vi "Match_Linear.vi"(0 "환산단위(보정값)":string, 3 "절대값?":bool, 4 "기준기명":string, 5 "교정(T) 보정(F)":bool=TRUE, 6 "열팽창계수(etc)":string="0", 7 "0보다 작음?":bool, 8 "환산단위(불확도)":string="μm", 9 "Cal STD in":string[][](array[string]), 10 "환산단위(교정값)":string, 11 "Condition Default":string[][](array[string])) -> (1 "Cal STD out":string[][](array[string]), 2 "Data out":string[][](array[string]))   [LabVIEW 2020]
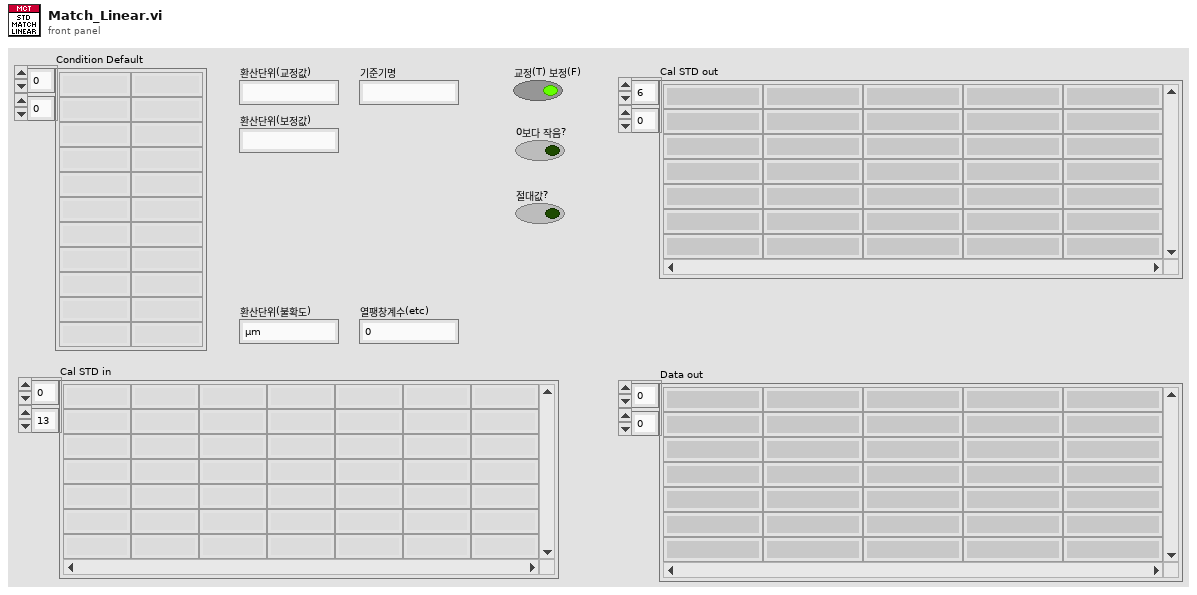
[diagram p1: front panel]
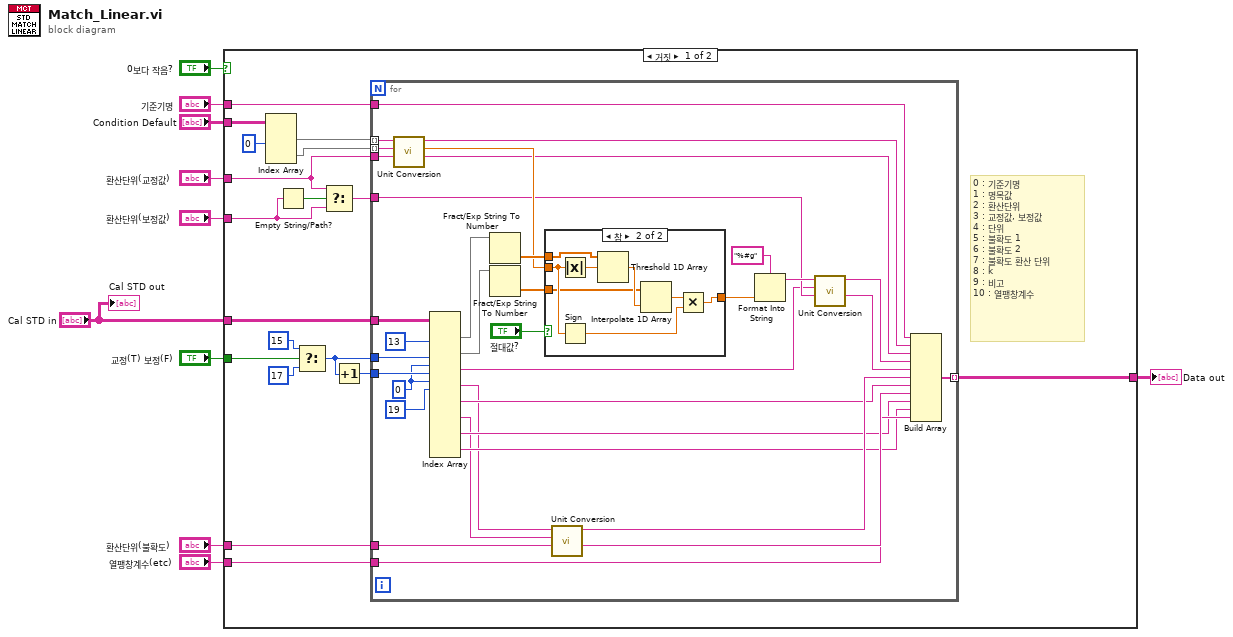
[diagram p0: block diagram]
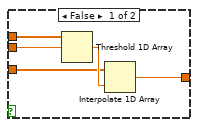
[diagram p2: hidden frame]
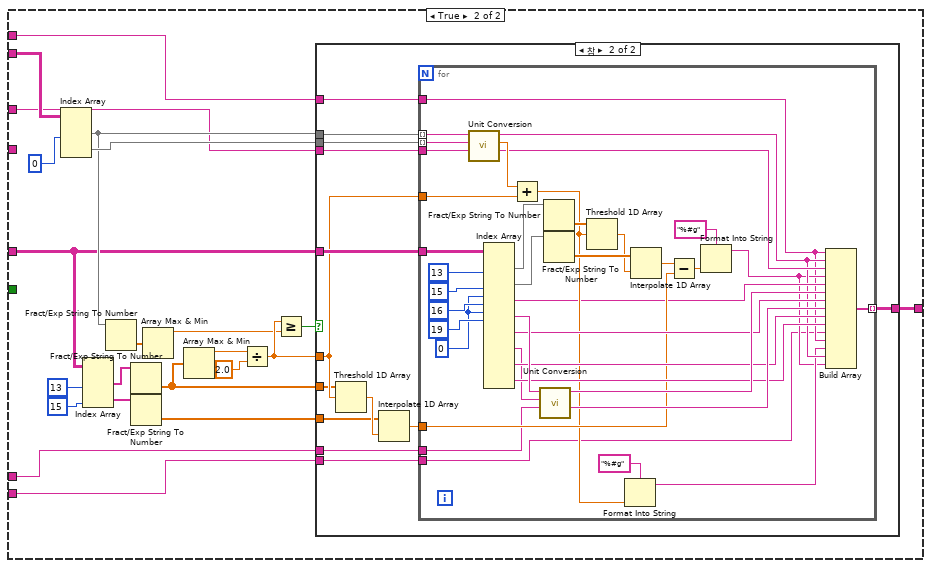
[diagram p3: hidden frame]
diagram:
  n1 = case shown="거짓" "0보다 작음?" {
    tunnel: "기준기명" -> [w28 w85]
    tunnel: "Cal STD in" -> [w27 w78]
    tunnel: "환산단위(교정값)" -> [w13 w77]
    tunnel: [w26 w88] -> w8
    tunnel: "환산단위(불확도)" -> [w25 w80]
    tunnel: "열팽창계수(etc)" -> [w24 w79]
    tunnel: "교정(T) 보정(F)" -> [w23 _]
    tunnel: "Condition Default" -> [w17 w81]
    tunnel: "환산단위(보정값)" -> [w12 _]
    frame False {
      # "0 : 기준기명\n1 : 명목값\n2 : 환산단위\n3 : 교정값, 보정값\n4 : 단위\n5 : 불확도 1\n6 : 불확도 2\n7 : 불확도 환산 단위\n8 : k\n9 : 비고\n10 : 열팽창계수"
      n2 = Index Array(array=w17, index (col) #1=0 ("비활성화된 인덱스 (열)")) -> (element #1=w16:string[], element #2=w15:string[])  [unwired: 3 in]
      n3 = Empty String/Path?(string/path=w12) -> (empty?=w14:bool)
      n4 = Select(t=15 ("인덱스 (행)"), s=w23, f=17 ("인덱스 (행)")) -> (s? t:f=w20:i32)
      n5 = Select(t=w13, s=w14, f=w12) -> (s? t:f=w11:string)
      n6 = Increment(x=w20) -> (x+1=w19:i32)
      n7 = for {
        tunnel: w27 -> [w63]
        tunnel: w16 -> [w57] mode=indexing
        tunnel: [w62] -> w26 mode=indexing
        tunnel: w15 -> [w56] mode=indexing
        tunnel: w13 -> [w55]
        tunnel: w25 -> [w54]
        tunnel: w28 -> [w53]
        tunnel: w24 -> [w48]
        tunnel: w20 -> [w45]
        tunnel: w19 -> [w44]
        tunnel: w11 -> [w31]
        w43 = 0 ("인덱스 (열)")
        n8 = call "Unit Conversion.vi"("환산단위"=w55, "입력단위"=w56, "입력값"=w57) -> ("환산단위"=w32:string, "환산값 (DBL)"=w60:dbl, "환산값 (string)"=w52:string)  [unwired: 3 in, 3 out]
        n9 = Index Array(array=w63, index (col) #1=13 ("인덱스 (행)"), index (col) #2=w45, index (row) #3=w43, index (col) #3=w44, index (row) #4=w43, index (col) #4=19 ("비활성화된 인덱스 (열)")) -> (element #1=w58:string[], element #2=w40:string[], element #3=w30:string, element #4=w36:string, element #5=w50:string, element #6=w35:string, element #7=w47:string, element #8=w46:string)  [unwired: 10 in]
        n10 = Fract/Exp String To Number(string=w58) -> (number=w61:dbl[])  [unwired: 3 in, 1 out]
        n11 = Fract/Exp String To Number(string=w40) -> (number=w39:dbl[])  [unwired: 3 in, 1 out]
        n12 = case shown="참" "절대값?" {
          tunnel: w61 -> [w68 w71]
          tunnel: w60 -> [w66 w72]
          tunnel: w39 -> [w65 w70]
          tunnel: [w64 w69] -> w37
          frame False {
            n13 = Threshold 1D Array(2:w66, 3:w68) -> (0:w67:dbl)  [unwired: 1 in]
            n14 = Interpolate 1D Array(1:w67, 2:w65) -> (0:w64:dbl)
          }
          frame True {
            n15 = Absolute Value(x=w72) -> (abs(x)=w76:dbl)
            n16 = Sign(1:w72) -> (0:w75:dbl)
            n17 = Threshold 1D Array(2:w76, 3:w71) -> (0:w74:dbl)  [unwired: 1 in]
            n18 = Interpolate 1D Array(1:w74, 2:w70) -> (0:w73:dbl)
            n19 = Multiply(x=w73, y=w75) -> (x*y=w69:dbl)
          }
        }
        n20 = call "Unit Conversion.vi"("환산단위"=w54, "입력단위"=w35, "입력값"=w36) -> ("환산단위"=w49:string, "환산값 (string)"=w51:string)  [unwired: 3 in, 4 out]
        n21 = Format Into String(format string="%#g" ("포맷 문자열"), w37) -> (resulting string=w34:string)  [unwired: 2 in, 1 out]
        n22 = call "Unit Conversion.vi"("환산단위"=w31, "입력단위"=w30, "입력값"=w34) -> ("환산단위"=w29:string, "환산값 (string)"=w33:string)  [unwired: 3 in, 4 out]
        n23 = Build Array(w53, w52, w32, w33, w29, w51, w50, w49, w47, w46, w48) -> (w62:string[])
      }
    }
    frame True {
      n24 = Index Array(array=w81, index (col) #1=0 ("비활성화된 인덱스 (열)")) -> (element #1=w82:string[], element #2=w83:string[])  [unwired: 3 in]
      n25 = Index Array(array=w78, index (col) #1=13 ("인덱스 (행)"), index (col) #2=15 ("인덱스 (행)")) -> (element #1=w91:string[], element #2=w92:string[])  [unwired: 2 in]
      n26 = Fract/Exp String To Number(string=w82) -> (number=w87:dbl[])  [unwired: 3 in, 1 out]
      n27 = Fract/Exp String To Number(string=w91) -> (number=w94:dbl[])  [unwired: 3 in, 1 out]
      n28 = Fract/Exp String To Number(string=w92) -> (number=w93:dbl[])  [unwired: 3 in, 1 out]
      n29 = Array Max & Min(array=w87) -> (max value=w86:dbl)  [unwired: 3 out]
      n30 = Array Max & Min(array=w94) -> (max value=w95:dbl)  [unwired: 3 out]
      n31 = Divide(x=w95, y=2.0) -> (x/y=w98:dbl)
      n32 = Greater Or Equal?(x=w98, y=w86) -> (x >= y?=w97:bool)
      n33 = case shown="참" w97 {
        tunnel: [_ w111] -> w88
        tunnel: w83 -> [_ w110]
        tunnel: w82 -> [_ w109]
        tunnel: w78 -> [_ w108]
        tunnel: w93 -> [_ w106]
        tunnel: w98 -> [_ w105]
        tunnel: w94 -> [_ w103]
        tunnel: w77 -> [_ w102]
        tunnel: w85 -> [_ w101]
        tunnel: w80 -> [_ w100]
        tunnel: w79 -> [_ w99]
        frame False {
        }
        frame True {
          n34 = Threshold 1D Array(2:w105, 3:w103) -> (0:w107:dbl)  [unwired: 1 in]
          n35 = Interpolate 1D Array(1:w107, 2:w106) -> (0:w104:dbl)
          n36 = for {
            tunnel: w108 -> [w149]
            tunnel: w109 -> [w146] mode=indexing
            tunnel: w110 -> [w145] mode=indexing
            tunnel: [w144] -> w111 mode=indexing
            tunnel: w105 -> [w131]
            tunnel: w104 -> [w129]
            tunnel: w102 -> [w125]
            tunnel: w101 -> [w114]
            tunnel: w100 -> [w113]
            tunnel: w99 -> [w112]
            w119 = 0 ("인덱스 (열)")
            n37 = call "Unit Conversion.vi"("환산단위"=w125, "입력단위"=w145, "입력값"=w146) -> ("환산단위"=w126:string, "환산값 (DBL)"=w139:dbl, "환산값 (string)"=w117:string)  [unwired: 3 in, 3 out]
            n38 = Index Array(array=w149, index (col) #1=13 ("인덱스 (행)"), index (col) #2=15 ("인덱스 (행)"), index (row) #3=w119, index (col) #3=16 ("인덱스 (행)"), index (row) #4=w119, index (col) #4=19 ("인덱스 (열)")) -> (element #1=w123:string[], element #2=w121:string[], element #3=w118:string, element #4=w141:string, element #5=w132:string, element #6=w133:string, element #7=w134:string, element #8=w135:string)  [unwired: 10 in]
            n39 = Add(x=w139, y=w131) -> (x+y=w127:dbl)
            n40 = call "Unit Conversion.vi"("환산단위"=w113, "입력단위"=w133, "입력값"=w141) -> ("환산단위"=w136:string, "환산값 (string)"=w137:string)  [unwired: 3 in, 4 out]
            n41 = Fract/Exp String To Number(string=w123) -> (number=w143:dbl[])  [unwired: 3 in, 1 out]
            n42 = Fract/Exp String To Number(string=w121) -> (number=w148:dbl[])  [unwired: 3 in, 1 out]
            n43 = Threshold 1D Array(2:w127, 3:w143) -> (0:w140:dbl)  [unwired: 1 in]
            n44 = Format Into String(format string="%#g" ("포맷 문자열"), w127) -> (resulting string=w116:string)  [unwired: 2 in, 1 out]
            n45 = Interpolate 1D Array(1:w140, 2:w148) -> (0:w147:dbl)
            n46 = Subtract(x=w147, y=w129) -> (x-y=w130:dbl)
            n47 = Format Into String(format string="%#g" ("포맷 문자열"), w130) -> (resulting string=w115:string)  [unwired: 2 in, 1 out]
            n48 = Build Array(w114, w117, w126, w115, w118, w137, w132, w136, w134, w135, w112, w114, w116, w117, w115) -> (w144:string[])
          }
        }
      }
    }
  }
  "Data out" <- w8
  "Cal STD out" <- "Cal STD in"
